vi "RegisterWindowsMessage.vi"(5 "RegisterWindowMessage":string) -> (2 "Message":u32 format="%.0x")   [LabVIEW 2011]
uses:
  user32.dll
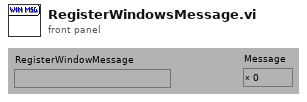
[diagram p1: front panel]
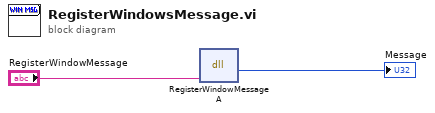
[diagram p0: block diagram]
diagram:
  n1 = dll-call lib="User32.dll" fn="RegisterWindowMessageA"("lpMessageString"="RegisterWindowMessage") -> ("dwMessageId"=→"Message":u32)  [unwired: 4 in, 2 out]
